vi "Configuration to Tree Items.vi"(8 "error in (no error)":errorcluster, 11 "Refnum In":T1) -> (0 "error out":errorcluster, 2 "Items":T2(array[cluster]), 3 "Refnum out":T1)   [LabVIEW 2017]
uses:
  DSF Configuration API/1.0.0/Public/Controls/DSF Config Data RefNum.ctl
  DSF Configuration API/1.0.0/DSF Configuration API.lvlib
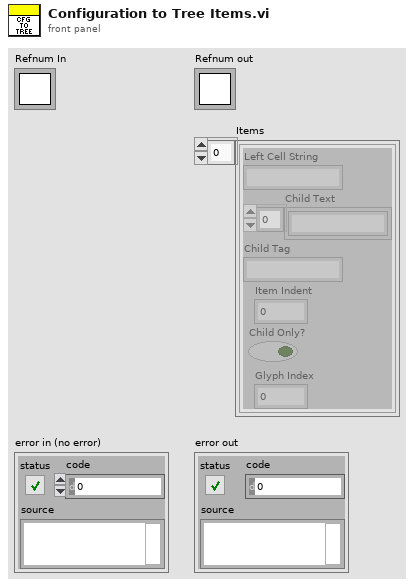
[diagram p1: front panel]
types:
  T1 = typedef "DSF Configuration API.lvlib/DSF Config Data RefNum.ctl" = refnum<k1>
  T2 = cluster{"Left Cell String":string, "Child Text":string[], "Child Tag":string, "Item Indent":i32, "Child Only?":bool, "Glyph Index":i32}[]
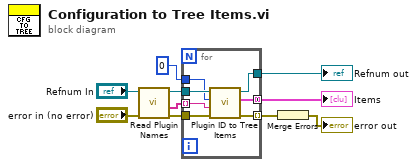
[diagram p0: block diagram]
diagram:
  n1 = call "Read Plugin Names.vi"("error in (no error)"="error in (no error)", "refnum"="Refnum In") -> ("error out"=w5:errorcluster, "names"=w6:string[], "refnum out"=w4:T1)  [unwired: 7 in]
  n2 = for {
    tunnel: w4 -> [w17]
    tunnel: w5 -> [w16]
    tunnel: w6 -> [w14] mode=indexing
    tunnel: [w15] -> w7 mode=indexing
    tunnel: 0 -> [w13]
    tunnel: [w12] -> w9 mode=concatenating
    tunnel: [w11] -> w10
    n3 = call "Plugin ID to Tree Items.vi"("error in (no error)"=w16, "Plugin ID"=w14, "Indent"=w13, "Refnum in"=w17) -> ("error out"=w15:errorcluster, "Items"=w12:T2, "Refnum out"=w11:T1)  [unwired: 5 in]
  }
  "Refnum out" <- w10
  "Items" <- w9
  n4 = Merge Errors(w7) -> (→"error out":errorcluster)
